vi "ray_intersect.vi"(8 "Distance":dbl, 9 "Direction":dbl[](array[numeric]), 10 "Origin":dbl[](array[numeric]), 11 "Sphere":T1) -> (0 "Distance":dbl, 3 "RayIntersect":bool)   [LabVIEW 2015]
uses:
  Sphere.ctl
  Material.ctl
  <vilib>/Analysis/baseanly.llb/Real Dot Product.vi
  <vilib>/Analysis/NI_AALBase.lvlib
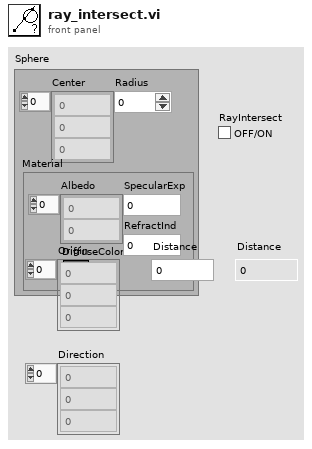
[diagram p1: front panel]
types:
  T1 = typedef "Sphere.ctl" = cluster{"Center":dbl[], "Radius":dbl, "Material":T2}
  T2 = typedef "Material.ctl" = cluster{"Albedo":dbl[], "DiffuseColor":u32, "SpecularExp":dbl, "RefractInd":dbl}
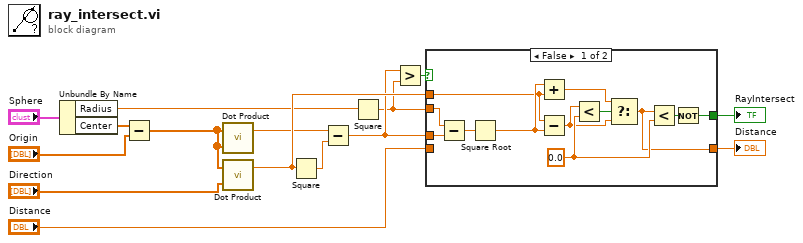
[diagram p0: block diagram]
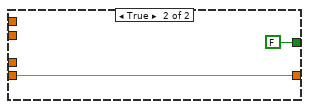
[diagram p2: hidden frame]
diagram:
  n1 = Unbundle By Name("Sphere") -> ("Radius"=w8:dbl, "Center"=w4:dbl[])
  n2 = Subtract(x=w4, y="Origin") -> (x-y=w9:dbl[])
  n3 = call-poly <vilib>:"Dot Product.vi"("Y Vector"=w9, "X Vector"=w9) -> ("X * Y"=w10:dbl)  [unwired: 1 out]
  n4 = call-poly <vilib>:"Dot Product.vi"("Y Vector"="Direction", "X Vector"=w9) -> ("X * Y"=w14:dbl)  [unwired: 1 out]
  n5 = Square(x=w14) -> (x^2=w7:dbl)
  n6 = Subtract(x=w10, y=w7) -> (x-y=w13:dbl)
  n7 = Square(x=w8) -> (x^2=w12:dbl)
  n8 = Greater?(x=w13, y=w12) -> (0:w11:bool)
  n9 = case shown="False" w11 {
    tunnel: [w17 FALSE] -> w15
    tunnel: w12 -> [w27 _]
    tunnel: w13 -> [w26 _]
    tunnel: w14 -> [w23 _]
    tunnel: [w16 w28] -> w2
    tunnel: "Distance" -> [_ w28]
    frame False {
      w21 = 0.0 ("y")
      n10 = Subtract(x=w27, y=w26) -> (x-y=w25:dbl)
      n11 = Square Root(x=w25) -> (sqrt(x)=w24:dbl)
      n12 = Add(x=w24, y=w23) -> (x+y=w20:dbl)
      n13 = Subtract(x=w23, y=w24) -> (x-y=w19:dbl)
      n14 = Less?(x=w19, y=w21) -> (x < y?=w22:bool)
      n15 = Select(t=w20, s=w22, f=w19) -> (s? t:f=w16:dbl)
      n16 = Less?(x=w16, y=w21) -> (x < y?=w18:bool)
      n17 = Not(x=w18) -> (.not. x?=w17:bool)
    }
    frame True {
    }
  }
  "RayIntersect" <- w15
  "Distance" <- w2
